vi "停止整机测试(子VI).vi"   [LabVIEW 2016]
types:
  T1 = cluster{"命令":string, cluster{"starting address":u16, "holding register value":u16}}
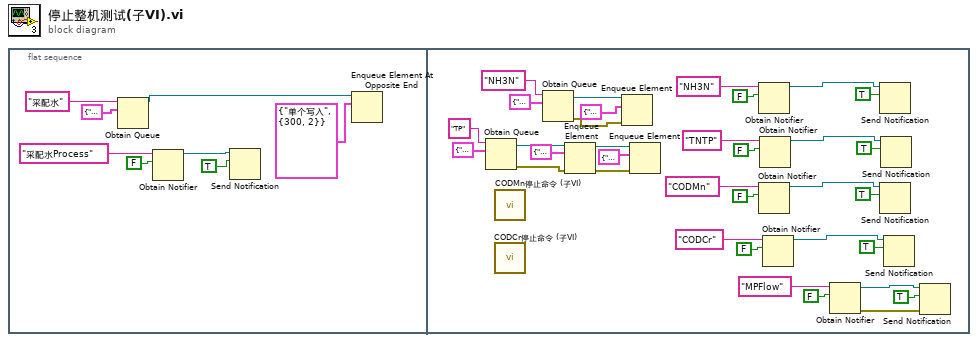
[diagram p0: block diagram]
diagram:
  n1 = flat-sequence {
    frame #0 {
      n2 = Obtain Queue(name (unnamed)="采配水" ("名称（未命名）"), element data type=cluster{"命令":string, "数据":variant} {"命令"="", "数据"=variant}) -> (queue out=w6:refnum<queue>)  [unwired: 3 in, 2 out]
      n3 = Obtain Notifier(name (unnamed)="采配水Process" ("名称（未命名）"), notification data type=FALSE) -> (notifier out=w8:refnum<notifier>)  [unwired: 2 in, 2 out]
      n4 = Send Notification(notification=TRUE ("通知"), notifier=w8) -> ()  [unwired: 1 in, 2 out]
      n5 = Enqueue Element At Opposite End(queue=w6, element=T1 {"命令"="单个写入", {"starting address"=300, "holding register value"=2}} ("元素")) -> ()  [unwired: 2 in, 3 out]
    }
    frame #1 {
      n6 = Obtain Queue(name (unnamed)="TP" ("名称（未命名）"), element data type=cluster{"命令":string, "data":variant} {"命令"="", "data"=variant}) -> (queue out=w35:refnum<queue>, error out=w10:errorcluster)  [unwired: 3 in, 1 out]
      n7 = call "CODMn停止命令 (子VI).vi"() -> ()  [unwired: 12 in]
      n8 = call "CODCr停止命令 (子VI).vi"() -> ()  [unwired: 12 in]
      n9 = Obtain Queue(name (unnamed)="NH3N" ("名称（未命名）"), element data type=cluster{"命令":string, "data":variant} {"命令"="", "data"=variant}) -> (queue out=w42:refnum<queue>, error out=w9:errorcluster)  [unwired: 3 in, 1 out]
      n10 = Enqueue Element(queue=w35, element=cluster{"命令":string, "data":variant} {"命令"="启动", "data"=variant(cluster{"站号":u16, "控制命令输出":u16[]} {"站号"=1, "控制命令输出"=[2816]})} ("元素"), error in (no error)=w10) -> (queue out=w13:refnum<queue>, error out=w11:errorcluster)  [unwired: 1 in, 1 out]
      n11 = Enqueue Element(queue=w42, element=cluster{"命令":string, "data":variant} {"命令"="启动", "data"=variant(cluster{"站号":u16, "控制命令输出":u16[]} {"站号"=3, "控制命令输出"=[2816]})} ("启动命令"), error in (no error)=w9) -> ()  [unwired: 1 in, 3 out]
      n12 = Enqueue Element(queue=w13, element=cluster{"命令":string, "data":variant} {"命令"="启动", "data"=variant(cluster{"站号":u16, "控制命令输出":u16[]} {"站号"=2, "控制命令输出"=[2816]})} ("元素"), error in (no error)=w11) -> ()  [unwired: 1 in, 3 out]
      n13 = Obtain Notifier(name (unnamed)="NH3N" ("名称（未命名）"), notification data type=FALSE) -> (notifier out=w39:refnum<notifier>)  [unwired: 2 in, 2 out]
      n14 = Obtain Notifier(name (unnamed)="CODMn" ("名称（未命名）"), notification data type=FALSE) -> (notifier out=w24:refnum<notifier>)  [unwired: 2 in, 2 out]
      n15 = Obtain Notifier(name (unnamed)="TNTP" ("名称（未命名）"), notification data type=FALSE) -> (notifier out=w31:refnum<notifier>)  [unwired: 2 in, 2 out]
      n16 = Obtain Notifier(name (unnamed)="CODCr" ("名称（未命名）"), notification data type=FALSE) -> (notifier out=w18:refnum<notifier>)  [unwired: 2 in, 2 out]
      n17 = Obtain Notifier(name (unnamed)="MPFlow" ("名称（未命名）"), notification data type=FALSE) -> (notifier out=w20:refnum<notifier>, error out=w19:errorcluster)  [unwired: 2 in, 1 out]
      n18 = Send Notification(notification=TRUE ("通知"), notifier=w39) -> ()  [unwired: 1 in, 2 out]
      n19 = Send Notification(notification=TRUE ("通知"), notifier=w24) -> ()  [unwired: 1 in, 2 out]
      n20 = Send Notification(notification=TRUE ("通知"), notifier=w31) -> ()  [unwired: 1 in, 2 out]
      n21 = Send Notification(notification=TRUE ("通知"), notifier=w18) -> ()  [unwired: 1 in, 2 out]
      n22 = Send Notification(notification=TRUE ("通知"), notifier=w20, error in (no error)=w19) -> ()  [unwired: 2 out]
    }
  }
